vi "Servo MSMT Set RF Power.vi"(8 "error in (no error)":errorcluster, 10 "Step In":refnum<k7>, 11 "Servo to Compression in":refnum<class "Servo to Compression.lvclass">) -> (0 "error out":errorcluster, 2 "Step Out":refnum<k7>, 3 "Servo to Compression out":refnum<class "Servo to Compression.lvclass">)   [LabVIEW 2018, in "Servo to Compression.lvlib" / "Servo to Compression.lvclass"]
uses:
  Servo to Compression.lvclass
  C:/Sequence Automation/Plugins/Measurement Interface.lvlibp/Measurement Interface.lvclass
  Plugins/Measurement Interface.lvlibp/Private Methods/Measurement Parameters/Read Measurement Parameters.vi
  Plugins/String Database.lvlibp/String Database.lvclass
  Plugins/Measurements/Servo MSMT.lvlibp/Servo MSMT.lvclass
  Plugins/TestStand API Tools (TSAT).lvlibp/Step Actions/TSAT Step Actions.lvlib
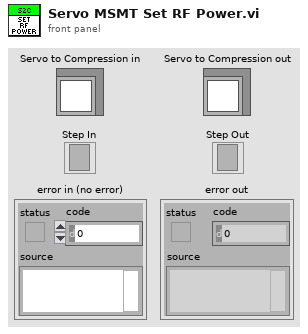
[diagram p1: front panel]
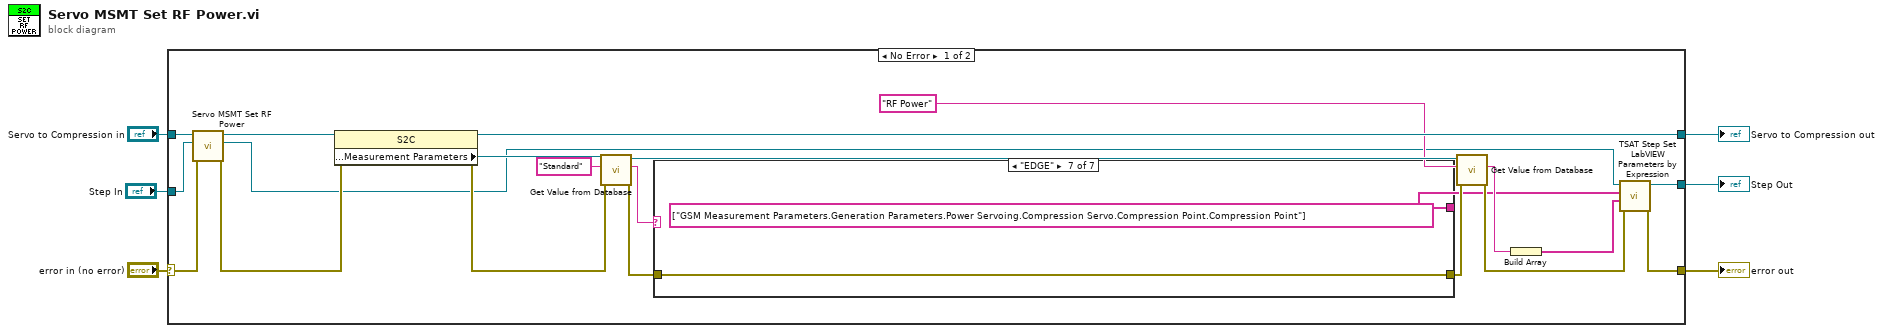
[diagram p0: block diagram]
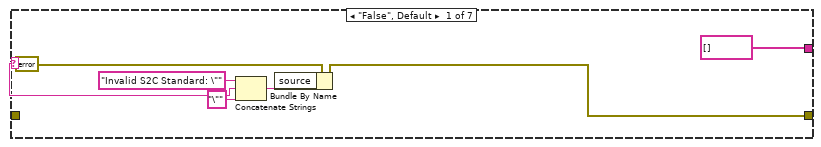
[diagram p2: hidden frame]
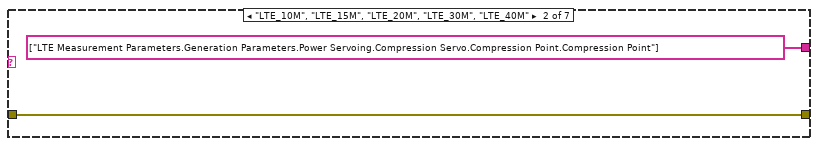
[diagram p3: hidden frame]
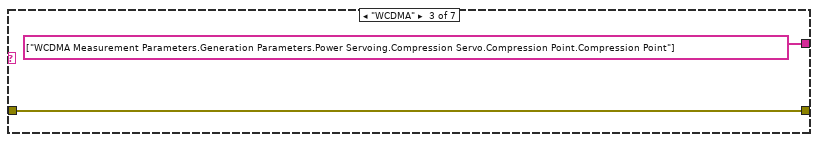
[diagram p4: hidden frame]
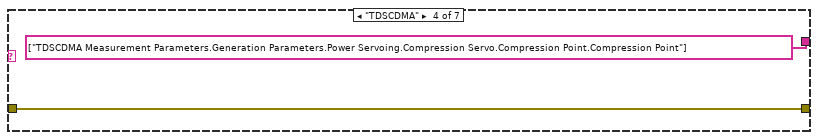
[diagram p5: hidden frame]
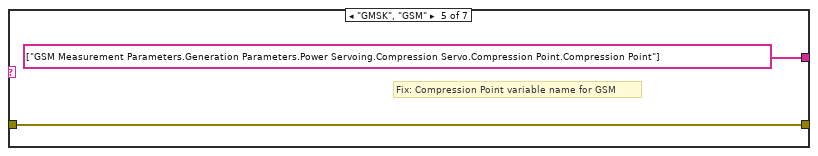
[diagram p6: hidden frame]
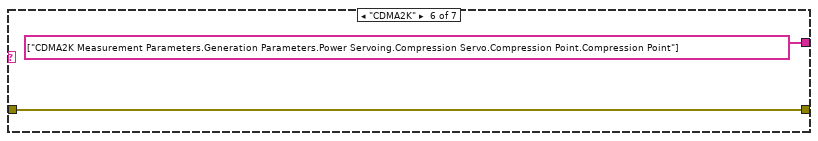
[diagram p7: hidden frame]
diagram:
  n1 = case shown="No Error" "error in (no error)" {
    selector: "error in (no error)" -> [w9 w49]
    tunnel: [w27 w48] -> w6
    tunnel: "Step In" -> [w8 w47]
    tunnel: [w21 w47] -> w4
    tunnel: [w20 w49] -> w3
    tunnel: "Servo to Compression in" -> [w11 w48]
    frame No Error {
      n2 = call-parent "Servo MSMT Set RF Power.vi"("error in (no error)"=w9, "Step In"=w8, "Servo MSMT in"=w11) -> ("error out"=w12:errorcluster, "Step Out"=w7:refnum<k7>, "Servo MSMT out"=w10:refnum<class "Servo to Compression.lvclass">)  [unwired: 6 in]
      n3 = property class="S2C"(reference=w10, error in=w12) -> (reference out=w27:refnum<class "Servo to Compression.lvclass">, error out=w25:errorcluster, "Protected Methods:Measurement Parameters"=w26:refnum<class "String Database.lvclass">)
      n4 = call "Get Value from Database.vi"("error in (no error)"=w25, "Entry Name"="Standard", "Message in"=w26) -> ("error out"=w17:errorcluster, "Entry Value"=w19:string, "Message out"=w23:refnum<class "String Database.lvclass">)  [unwired: 5 in, 1 out]
      n5 = case shown="\"EDGE\"" w19 {
        selector: w19 -> [w29 _ _ _ _ _ _]
        tunnel: [w32 w36 w38 w40 w42 w44 w46] -> w18
        tunnel: w17 -> [_ w36 w38 w40 w42 w44 w46]
        tunnel: [string[] [] string[] ["LTE Measurement Parameters.Generation Parameters.Power Servoing.Compression Servo.Compression Point.Compression Point"] string[] ["WCDMA Measurement Parameters.Generation Parameters.Power Servoing.Compression Servo.Compression Point.Compression Point"] string[] ["TDSCDMA Measurement Parameters.Generation Parameters.Power Servoing.Compression Servo.Compression Point.Compression Point"] string[] ["GSM Measurement Parameters.Generation Parameters.Power Servoing.Compression Servo.Compression Point.Compression Point"] string[] ["CDMA2K Measurement Parameters.Generation Parameters.Power Servoing.Compression Servo.Compression Point.Compression Point"] string[] ["GSM Measurement Parameters.Generation Parameters.Power Servoing.Compression Servo.Compression Point.Compression Point"]] -> w13
        frame "False", Default {
          n6 = Concatenate Strings("Invalid S2C Standard: \"" ("source"), w29, "\"" ("string")) -> (w30:string)
          n7 = Bundle By Name(cluster=errorcluster {"status"=TRUE, "code"=9988, "source"=""} ("error out"), "source"=w30) -> (w32:errorcluster)
        }
        frame "LTE_10M", "LTE_15M", "LTE_20M", "LTE_30M", "LTE_40M" {
        }
        frame "WCDMA" {
        }
        frame "TDSCDMA" {
        }
        frame "GMSK", "GSM" {
          # "Fix: Compression Point variable name for GSM"
        }
        frame "CDMA2K" {
        }
        frame "EDGE" {
        }
      }
      n8 = call "Get Value from Database.vi"("error in (no error)"=w18, "Entry Name"="RF Power", "Message in"=w23) -> ("error out"=w16:errorcluster, "Entry Value"=w15:string)  [unwired: 5 in, 2 out]
      n9 = Build Array(w15) -> (w14:string[])
      n10 = call "TSAT Step Set LabVIEW Parameters by Expression.vi"("Error In"=w16, "Value Expressions"=w14, "Parameters to Set"=w13, "Step In"=w7) -> ("Error Out"=w20:errorcluster, "Step Out"=w21:refnum<k7>)  [unwired: 6 in]
    }
    frame Error {
    }
  }
  "error out" <- w3
  "Servo to Compression out" <- w6
  "Step Out" <- w4
